vi "soundParametersRef.vi"(4 "Sound Parameters":refnum<vi>, 7 "Sound Device IN":T3 {"task ID" format="%.0x"}) -> (0 "#samples":u32, 2 "En funcionamiento?":bool, 3 "Sound Device OUT":T3 {"task ID" format="%.0x"})   [LabVIEW 2010]
uses:
  <vilib>/sound2/lvsound2.llb/Sound Output Task ID.ctl
  <vilib>/sound2/lvsound2.llb/Sound Data Format.ctl
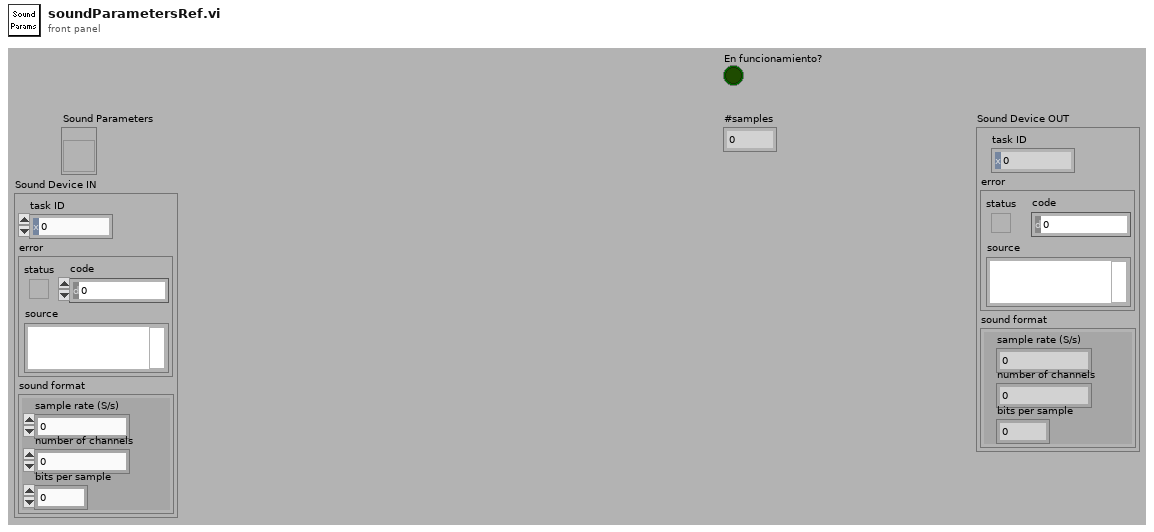
[diagram p1: front panel]
types:
  T1 = typedef "Sound Output Task ID.ctl" = u32
  T2 = typedef "Sound Data Format.ctl" = cluster{"sample rate (S/s)":dbl, "number of channels":i32, "bits per sample":i32}
  T3 = cluster{"task ID":T1, "error":errorcluster, "sound format":T2}
  T4 = cluster{"time (ms)":dbl, "sound format":T2, "device ID":u32}
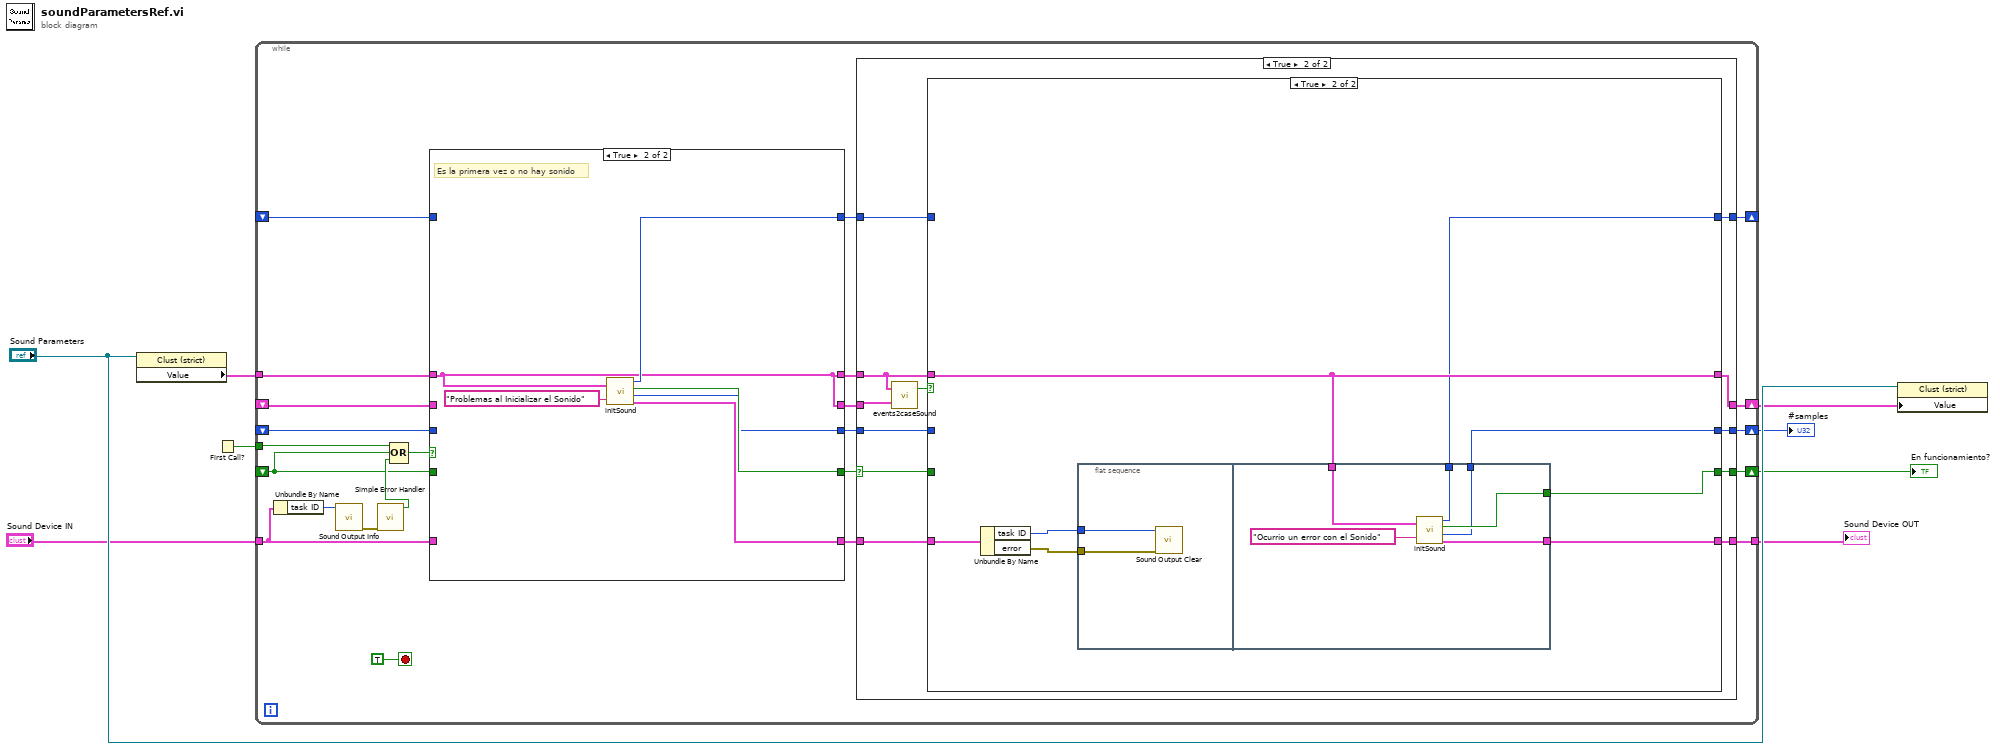
[diagram p0: block diagram]
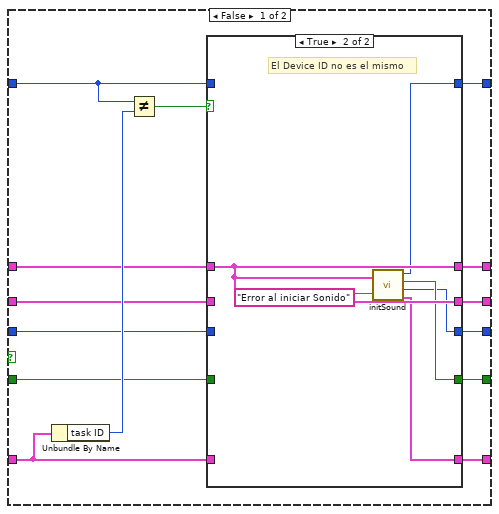
[diagram p4: hidden frame]
diagram:
  n1 = property class="Clust (strict)"(reference="Sound Parameters") -> ("Value"=w7:T4)  [unwired: 1 in, 2 out]
  n2 = First Call?() -> (First Call?: T/F=w8:bool)
  n3 = while {
    tunnel: w7 -> [w27]
    shift-right: [w30] -> w5
    shift-left: _ -> [w26]
    tunnel: "Sound Device IN" -> [w18]
    tunnel: [w29] -> w3
    tunnel: w8 -> [w19]
    shift-right: [w20] -> _
    shift-left: _ -> [w23]
    shift-right: [w9] -> w1
    shift-left: _ -> [w14]
    shift-right: [w13] -> w2
    shift-left: _ -> [w11]
    stop <- TRUE stop-if-true
    n4 = Unbundle By Name(w18) -> ("task ID"=w17:T1)
    n5 = call <vilib>:"Sound Output Info.vi"("task ID"=w17) -> ("error out"=w16:errorcluster)  [unwired: 7 in, 3 out]
    n6 = call <vilib>:"Simple Error Handler.vi"("error in (no error)"=w16) -> ("error?"=w15:bool)  [unwired: 4 in, 4 out]
    n7 = Compound Arithmetic op=OR(w19, w14, w15) -> (w22:bool)
    n8 = case shown="True" w22 {
      tunnel: [w76 w100] -> w21
      tunnel: [w78 w98] -> w28
      tunnel: w27 -> [w79 w98]
      tunnel: w26 -> [w74 _]
      tunnel: [w77 w98] -> w25
      tunnel: [w83 w101] -> w24
      tunnel: w18 -> [w82 _]
      tunnel: w23 -> [w72 _]
      tunnel: [w75 w99] -> w10
      tunnel: w14 -> [w73 _]
      tunnel: [w71 w97] -> w12
      tunnel: w11 -> [w70 _]
      frame False {
        n9 = Unbundle By Name(w82) -> ("task ID"=w81:T1)
        n10 = Not Equal?(x=w72, y=w81) -> (x != y?=w80:bool)
        n11 = case shown="True" w80 {
          tunnel: [w89 w93] -> w83
          tunnel: w82 -> [w89 _]
          tunnel: w79 -> [w88 w95]
          tunnel: [w88 w95] -> w78
          tunnel: [w87 w95] -> w77
          tunnel: [w85 w94] -> w76
          tunnel: [w86 w92] -> w75
          tunnel: w74 -> [w87 _]
          tunnel: w73 -> [w86 _]
          tunnel: w72 -> [w85 _]
          tunnel: [w84 w91] -> w71
          tunnel: w70 -> [w84 _]
          frame False {
            # "Sigue siendo todo igual"
          }
          frame True {
            # "El Device ID no es el mismo"
            n12 = call "initSound.vi"("Error Message"="Error al iniciar Sonido", "Sound Parameters"=w95) -> ("Sound Device OUT"=w93:T3, "# samples"=w91:u32, "Inizializo?"=w92:bool, "task ID"=w94:T1)
          }
        }
      }
      frame True {
        # "Es la primera vez o no hay sonido"
        n13 = call "initSound.vi"("Error Message"="Problemas al Inicializar el Sonido", "Sound Parameters"=w98) -> ("Sound Device OUT"=w101:T3, "# samples"=w97:u32, "Inizializo?"=w99:bool, "task ID"=w100:T1)
      }
    }
    n14 = case shown="True" w10 {
      selector: w10 -> [w32 w37]
      tunnel: [w36 w47] -> w30
      tunnel: [w35 w46] -> w29
      tunnel: w21 -> [w34 w45]
      tunnel: w28 -> [w36 w42]
      tunnel: w25 -> [_ w41]
      tunnel: w24 -> [w35 w44]
      tunnel: [w34 w43] -> w20
      tunnel: [w33 w40] -> w13
      tunnel: w12 -> [w33 w39]
      tunnel: [w32 w38] -> w9
      frame False {
      }
      frame True {
        n15 = call "events2caseSound.vi"("Sound Controls Old"=w41, "Sound Controls New"=w42) -> ("Sound Cambio?"=w48:bool)  [unwired: 1 out]
        n16 = case shown="True" w48 {
          tunnel: [w53 w57] -> w47
          tunnel: w42 -> [w53 w57]
          tunnel: w44 -> [w52 w61]
          tunnel: [w52 w56] -> w46
          tunnel: w45 -> [w51 _]
          tunnel: [w51 w55] -> w43
          tunnel: [w50 w54] -> w40
          tunnel: w39 -> [w50 _]
          tunnel: [w49 w58] -> w38
          tunnel: w37 -> [w49 _]
          frame False {
          }
          frame True {
            n17 = Unbundle By Name(w61) -> ("task ID"=w59:T1, "error"=w60:errorcluster)
            n18 = flat-sequence {
              tunnel: w59 -> [w63]
              tunnel: w60 -> [w62]
              tunnel: [w67] -> w58
              tunnel: w57 -> [w69]
              tunnel: [w66] -> w56
              tunnel: [w65] -> w55
              tunnel: [w64] -> w54
              frame #0 {
                n19 = call <vilib>:"Sound Output Clear.vi"("error in (no error)"=w62, "task ID"=w63) -> ()  [unwired: 9 in, 1 out]
              }
              frame #1 {
                n20 = call "initSound.vi"("Error Message"="Ocurrio un error con el Sonido" ("message"), "Sound Parameters"=w69) -> ("Sound Device OUT"=w66:T3, "# samples"=w64:u32, "Inizializo?"=w67:bool, "task ID"=w65:T1)
              }
            }
          }
        }
      }
    }
  }
  "Sound Device OUT" <- w3
  "#samples" <- w2
  "En funcionamiento?" <- w1
  n21 = property class="Clust (strict)"(reference="Sound Parameters", "Value"=w5) -> ()  [unwired: 1 in, 2 out]
